vi "Search 2D Array (U32).vi"(10 "Element":u32, 11 "Array":u32[][](array[numeric])) -> (3 "Locations":i32[][](array[numeric]))   [LabVIEW 2020]
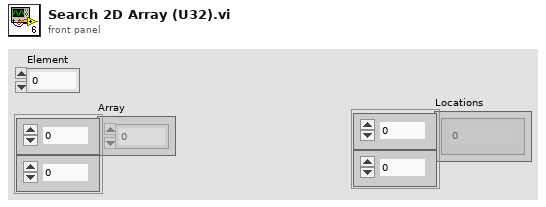
[diagram p1: front panel]
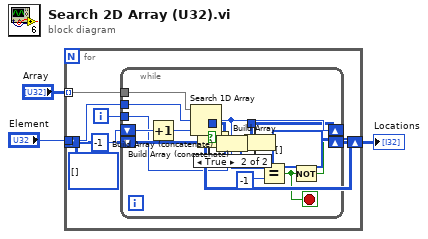
[diagram p0: block diagram]
diagram:
  n1 = for {
    tunnel: "Array" -> [w12] mode=indexing
    tunnel: "Element" -> [w11]
    shift-right: [w6] -> w2
    shift-left: i32[][] [] -> [w7]
    i -> [w10]
    n2 = while {
      tunnel: w12 -> [w24]
      tunnel: w11 -> [w23]
      shift-right: [w20] -> _
      shift-left: -1 ("index of element") -> [w22]
      tunnel: w10 -> [w19]
      shift-right: [w13] -> w9
      shift-left: i32[][] [] ("Array 2") -> [w14]
      stop <- w16 stop-if-true
      n3 = Increment(x=w22) -> (x+1=w17:i32)
      n4 = Search 1D Array(1D array=w24, element=w23, start index (0)=w17) -> (index of element=w20:i32)
      n5 = Build Array(w19, w20) -> (w18:i32[])
      n6 = Equal?(x=w20, y=-1) -> (x = y?=w16:bool)
      n7 = Not(x=w16) -> (.not. x?=w15:bool)
      n8 = case shown="True" w15 {
        tunnel: w14 -> [w25 w27]
        tunnel: w18 -> [_ w26]
        tunnel: [w25 w28] -> w13
        frame False {
        }
        frame True {
          n9 = Build Array (concatenate)(w27, w26) -> (w28:i32[][])
        }
      }
    }
    n10 = Build Array (concatenate)(w7, w9) -> (w6:i32[][])
  }
  "Locations" <- w2
